vi "finish_photon_stream.vi"(8 "error in (no error)":errorcluster, 11 "hydraharp in":refnum<class "hydraharp.lvclass">) -> (0 "error out":errorcluster, 3 "hydraharp out":refnum<class "hydraharp.lvclass">)   [LabVIEW 2015, in "hydraharp.lvclass"]
uses:
  hydraharp.lvclass
  hydraharp.lvclass/hydraharp.ctl
  hhlib.dll
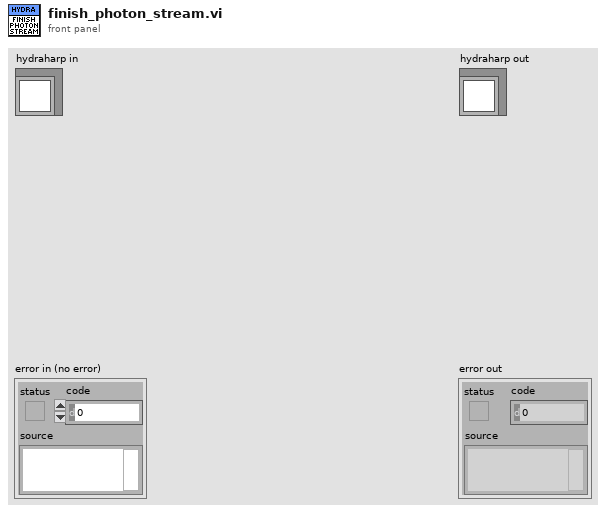
[diagram p1: front panel]
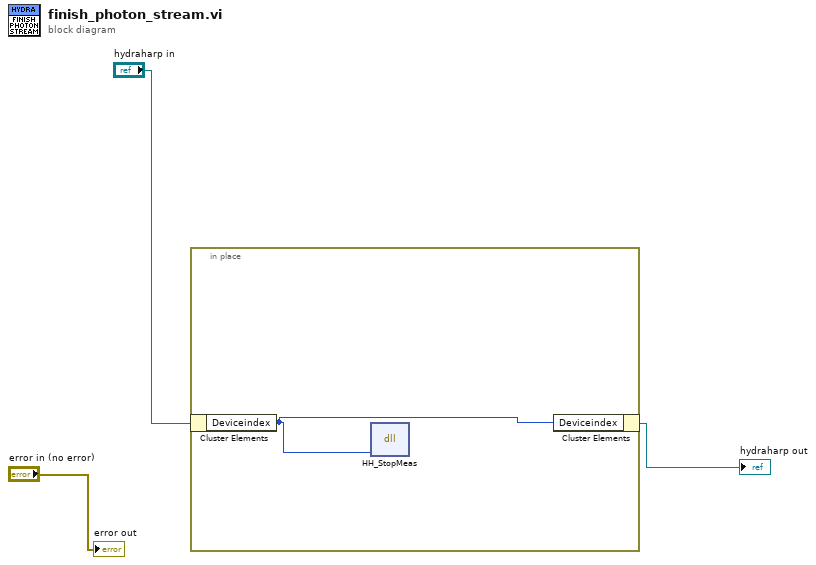
[diagram p0: block diagram]
diagram:
  n1 = in-place {
    n2 = in-place-cluster #1("hydraharp in") -> ("Deviceindex"=w4:i32)
    n3 = dll-call lib="hhlib.dll" fn="HH_StopMeas"("devidx"=w4) -> ()  [unwired: 5 in, 2 out]
    n4 = in-place-cluster #1("Deviceindex"=w4) -> (→"hydraharp out":refnum<class "hydraharp.lvclass">)
  }
  "error out" <- "error in (no error)"
